vi "makeDecisions.vi"(8 "error in (no error)":errorcluster, 10 "model":refnum<class "Model.lvclass">, 11 "WaitingForSettledSTState in":refnum<class "WaitingForSettledSTState.lvclass">) -> (0 "error out":errorcluster, 2 "model 2":refnum<class "Model.lvclass">, 3 "WaitingForSettledSTState out":refnum<class "WaitingForSettledSTState.lvclass">)   [LabVIEW 2015, in "WaitingForSettledSTState.lvclass"]
uses:
  WaitingForSettledSTState.lvclass
  Model/Model/Model.lvclass
  Typedefs/StateSelector.ctl
  TestingStiffnessState/TestingStiffnessState.lvclass
  Typedefs/M1M3SSSTypedefs.lvlib
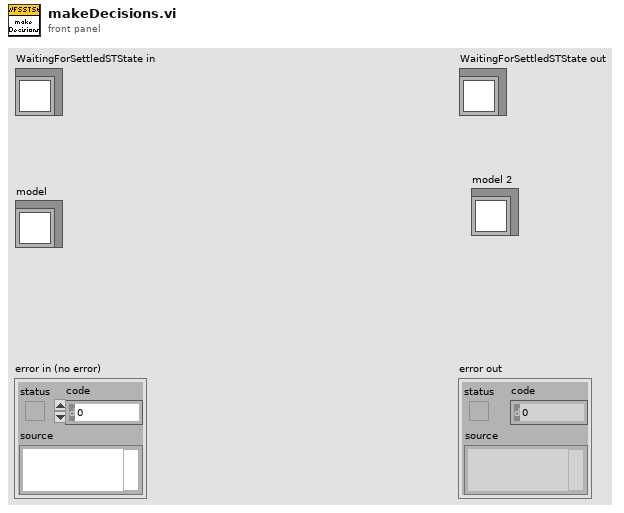
[diagram p1: front panel]
types:
  T1 = typedef "M1M3SSSTypedefs.lvlib/StateSelector.ctl" = enum16{"FaultState", "OffState", "RampingUpPressurePState", "RampingUpPressureSTState", "StandbyState", "StoppedState", "WaitingForSettledPState", "WaitingForSettledSTState"}
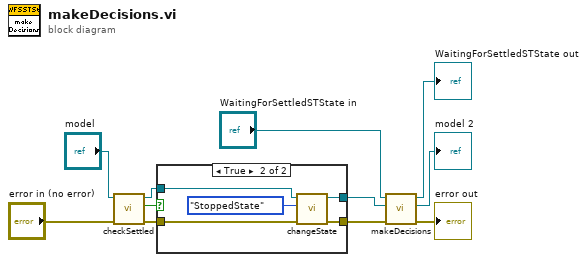
[diagram p0: block diagram]
diagram:
  n1 = call "checkSettled.vi"("error in (no error)"="error in (no error)", "Model in"="model") -> ("error out"=w7:errorcluster, "settledIsTrue"=w5:bool, "Model out"=w6:refnum<class "Model.lvclass">)  [unwired: 7 in]
  n2 = case shown="True" w5 {
    tunnel: [w13 w15] -> w2
    tunnel: w7 -> [w13 w16]
    tunnel: [w12 w17] -> w1
    tunnel: w6 -> [w12 w18]
    frame False {
    }
    frame True {
      n3 = call "changeState.vi"("error in (no error)"=w16, "State:"=StateSelector."StoppedState", "Model in"=w18) -> ("error out"=w15:errorcluster, "Model out"=w17:refnum<class "Model.lvclass">)  [unwired: 7 in]
    }
  }
  n4 = call-parent "makeDecisions.vi"("error in (no error)"=w2, "model"=w1, "EnabledState in"="WaitingForSettledSTState in") -> ("error out"=→"error out":errorcluster, "model 2"=→"model 2":refnum<class "Model.lvclass">, "EnabledState out"=→"WaitingForSettledSTState out":refnum<class "WaitingForSettledSTState.lvclass">)  [unwired: 6 in]
